vi "Stage Playback with send.vi"(8 "error in (no error)":errorcluster, 10 "IQ Swap Enabled":bool=TRUE, 11 "input cluster":T1={"Test_File"=path "", "Status"="Done", "RF_Center_Freq"=0.0, "RF_Gain"=0.0, "BB_Gain"=0.0, "Error 2"="", "file_max"=0, "file_index"=0}) -> (0 "error out":errorcluster, 2 "output cluster":T1={"Test_File"=path "", "Status"="Done", "RF_Center_Freq"=0.0, "RF_Gain"=0.0, "BB_Gain"=0.0, "Error 2"="", "file_max"=0, "file_index"=0}, 3 "Playback Progress":i32(slide)=383 scale=-1.0..536.0)   [LabVIEW 2017]
uses:
  TypeDef/ESC Internal Data Structure (types).ctl
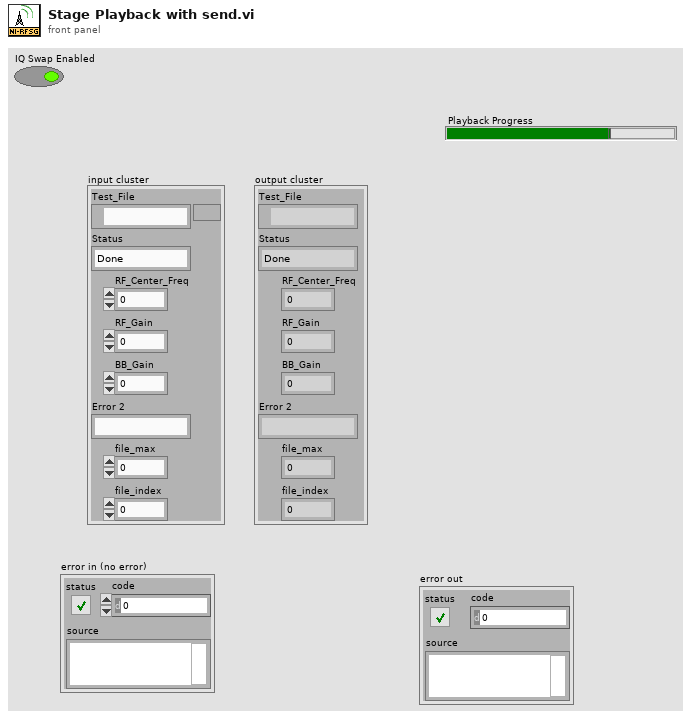
[diagram p1: front panel]
types:
  T1 = typedef "ESC Internal Data Structure (types).ctl" = cluster{"Test_File":path, "Status":string, "RF_Center_Freq":dbl, "RF_Gain":dbl, "BB_Gain":dbl, "Error 2":string, "file_max":u64, "file_index":u64}
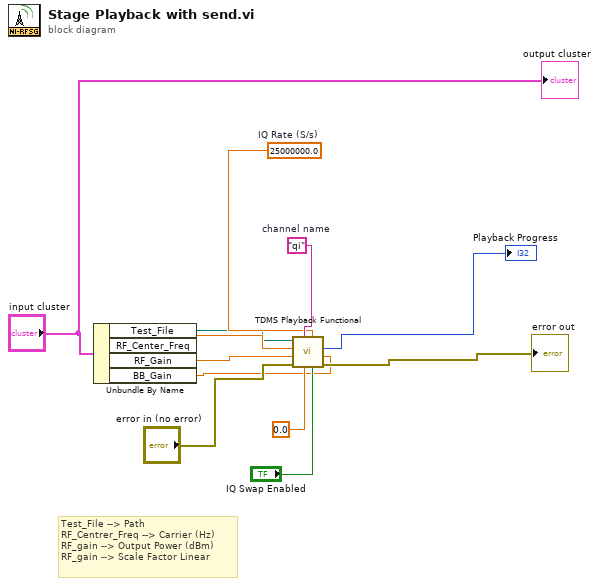
[diagram p0: block diagram]
diagram:
  w9 = 25000000.0  # IQ Rate (S/s)
  w10 = "qi"  # channel name
  # "Test_File --> Path\nRF_Centrer_Freq --> Carrier (Hz)\nRF_gain --> Output Power (dBm)\nRF_gain --> Scale Factor Linear"
  n1 = Unbundle By Name("input cluster") -> ("Test_File"=w4:path, "RF_Center_Freq"=w5:dbl, "RF_Gain"=w11:dbl, "BB_Gain"=w1:dbl)
  n2 = call "TDMS Playback Functional.vi"("Scale Factor Linear"=w1, "IQ Swap Enabled"="IQ Swap Enabled", "IQ Rate (S/s)"=w9, "pre filter gain"=0.0, "channel name (iq/qi)"=w10, "error in"="error in (no error)", "Output Power (dBm)"=w11, "Carrier (Hz)"=w5, "Path"=w4) -> ("error out"=→"error out":errorcluster, "Playback Progress"=→"Playback Progress":i32)  [unwired: 1 in]
  "output cluster" <- "input cluster"
